vi "Queue Decorate.vi"(10 "Queue Actor":refnum<class "Queue Actor.lvclass">, 11 "Base Queue Actor in":refnum<class "Base Queue Actor.lvclass">) -> (3 "Base Queue Actor out":refnum<class "Base Queue Actor.lvclass">)   [LabVIEW 2021, in "jettl.lvlib" / "Base Queue Actor.lvclass"]
uses:
  Base Queue Actor.lvclass
  Queue Actor/Queue Actor.lvclass
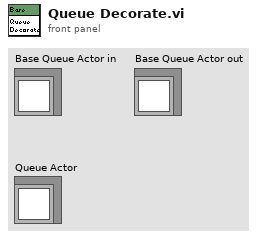
[diagram p1: front panel]
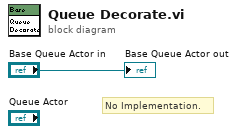
[diagram p0: block diagram]
diagram:
  # "No Implementation."
  "Base Queue Actor out" <- "Base Queue Actor in"
